vi "Test_ICR.vi"(8 "error in (no error)":errorcluster, 10 "ICR Queue":refnum<queue>, 11 "UI Queue":refnum<queue>) -> (0 "error out":errorcluster)   [LabVIEW 2017]
uses:
  controls/QMH_ICR_Message.ctl
  controls/QMH_ICR_Command.ctl
  controls/QMH_UI_Message.ctl
  controls/QMH_UI_Command.ctl
  controls/HARDWARE_Resources.ctl
  controls/PROCESSING_Inputs.ctl
  controls/QMH_ICR_Cluster.ctl
panel:
  out "Accum Name":string
  in  "PROCESSING  Inputs":T1={"Reference Mass"=300.0939, "Cyclotron Freq"=255.727, "Magnetron Freq"=0.001} caption="DATA Inputs" {"Magnetron Freq" format="%.5g"; "Cyclotron Freq" format="%.5g"; "Reference Mass" format="%.5g"}
  in  "Start":bool
  in  "Stop":bool
  in  "Send Trigger":bool
  out "Total Duration":i32
  out "Number of  Accumulations":i16
  out "Accumulation":i16
  in  "Use Software Trigger":bool=TRUE
  in  "Graph Chooser":T2(radio)=enum."Mass Spectrum"
  out "Remaining Time":string
  out "Spectrum Path":path
  out "Spectrum Prefix":string
  out "Spectrum Name":string
  out "Mass Accumulated":cluster{dbl[], dbl[]}(graph)
  out "Mass Spectrum":cluster{dbl[], dbl[]}(graph)
  out "Frequency Spectrum":cluster{dbl[], dbl[]}(graph)
  out "Signal":cluster{dbl[], dbl[]}(graph)
  in  "HARDWARE Resources":T3={"AO6711 Physical Channels"="Analog/ao0:3", "AO6711 Task Name"="", "AWG5421 Resource Name"="Waveform", "DIGIT 5122 Resource Name"="Digitizer", "HSDIO Resource Name"="Sequencer"}
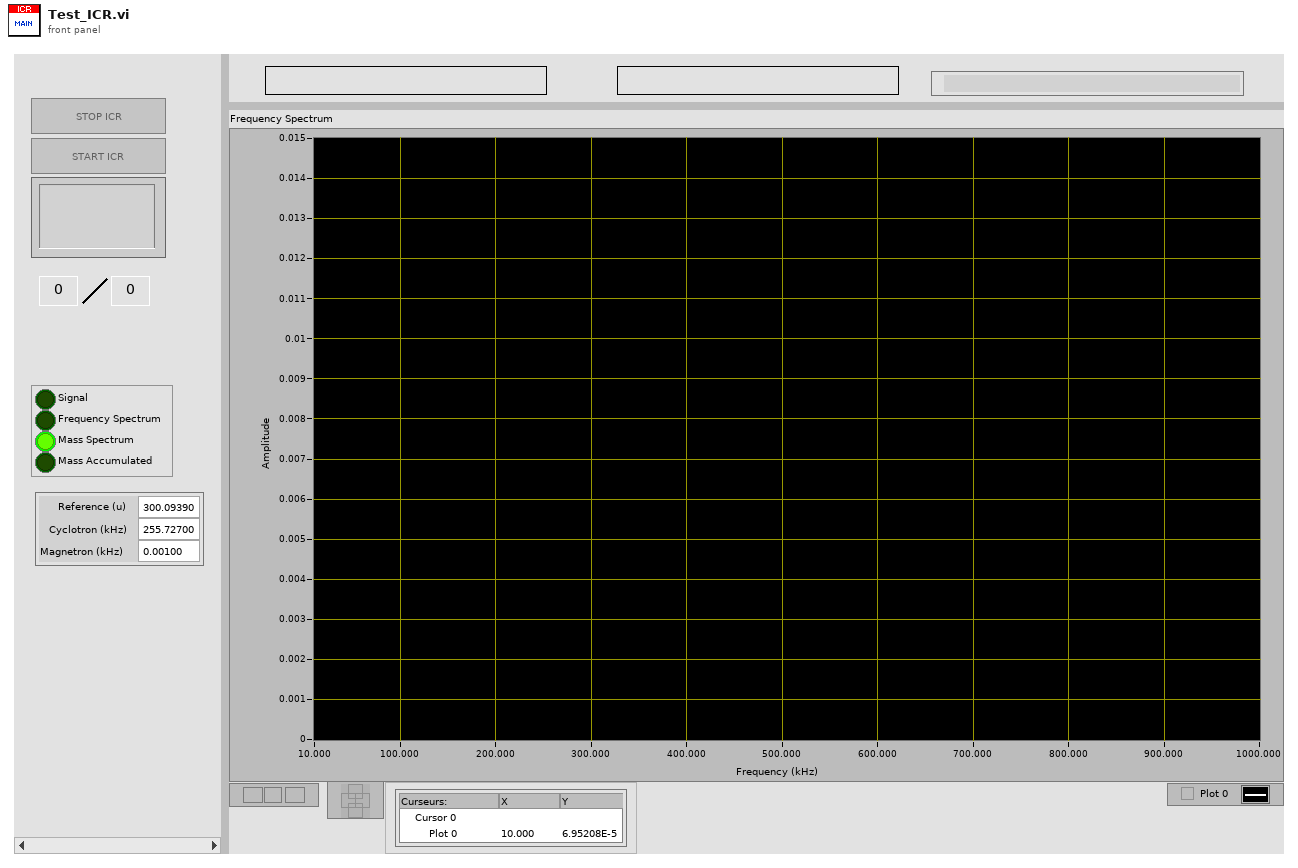
[diagram p1: front panel]
types:
  T1 = typedef "PROCESSING_Inputs.ctl" = cluster{"Reference Mass":dbl, "Cyclotron Freq":dbl, "Magnetron Freq":dbl}
  T2 = enum32{"Signal", "Frequency Spectrum", "Mass Spectrum", "Mass Accumulated"}
  T3 = typedef "HARDWARE_Resources.ctl" = cluster{"AO6711 Physical Channels":tag, "AO6711 Task Name":refnum<k21>, "AWG5421 Resource Name":refnum<k15>, "DIGIT 5122 Resource Name":refnum<k15>, "HSDIO Resource Name":refnum<k15>}
  T4 = typedef "QMH_ICR_Cluster.ctl" = cluster{"Use Software Trigger":refnum<vi>, "Send Trigger":refnum<vi>, "Stop":refnum<vi>, "Start":refnum<vi>, "HARDWARE Resources":refnum<vi>, "Total Duration":refnum<vi>, "Remaining Time":refnum<vi>, "Accumulation":refnum<vi>, "Number of  Accumulations":refnum<vi>, "Graph Chooser":refnum<vi>, "Signal":refnum<vi>, "Frequency Spectrum":refnum<vi>, "Mass Spectrum":refnum<vi>, "Mass Accumulated":refnum<vi>, "Processing":refnum<vi>, "Spectrum Path":refnum<vi>, "Spectrum Prefix":refnum<vi>, "Spectrum Name":refnum<vi>, "Accum Name":refnum<vi>, "Disk Writing Done":refnum<notifier>}
  T5 = typedef "QMH_ICR_Command.ctl" = enum16{"Initialize", "Sequence Setup", "ICR Start", "ICR Stop", "Hardware Setup", "Next Accumulation", "Waiting for Trigger", "Sequence Started", "Sequence Finished", "Writing Data", "Hardware Reset", "Exit"}
  T6 = typedef "QMH_UI_Command.ctl" = enum16{"Initialize", "UI Load", "UI Save", "UI Save As", "UI Change Experiment", "UI Change Voltages", "UI Change Sequence", "UI Change Expert", "Ready to Start", "UI Start", "Waiting for ICR", "UI Exit", "Update Report", "Update ICR Report"}
  T7 = typedef "QMH_ICR_Message.ctl" = cluster{"Command":T5, "Data":variant}
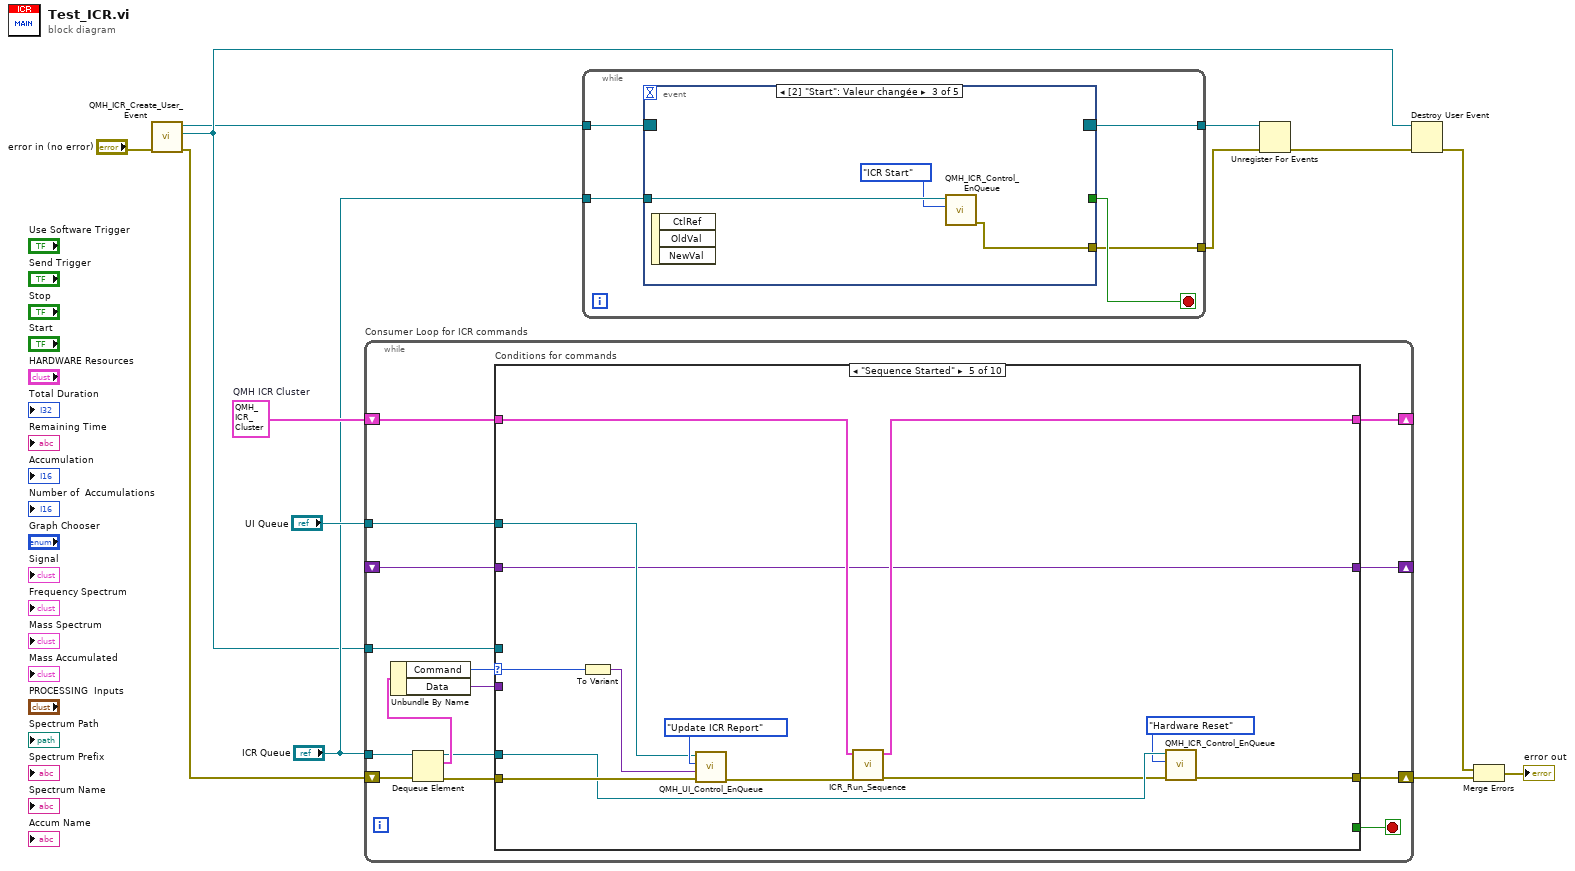
[diagram p0: block diagram]
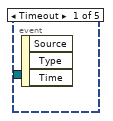
[diagram p2: hidden frame]
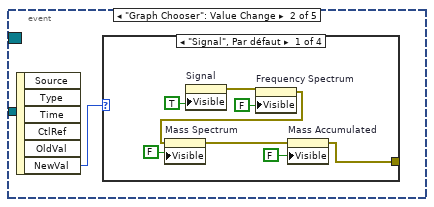
[diagram p3: hidden frame]
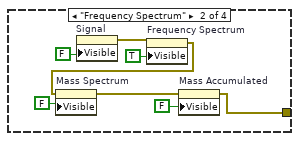
[diagram p4: hidden frame]
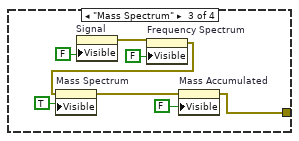
[diagram p5: hidden frame]
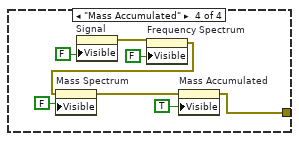
[diagram p6: hidden frame]
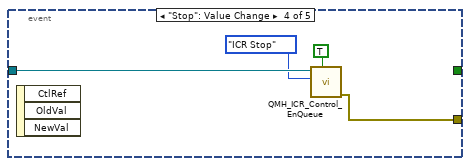
[diagram p7: hidden frame]
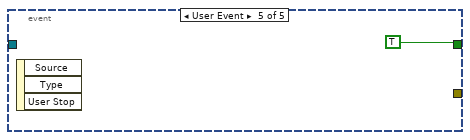
[diagram p8: hidden frame]
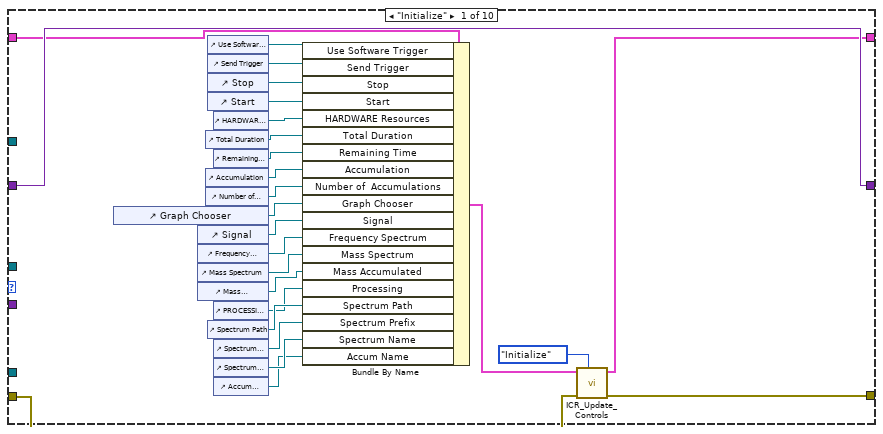
[diagram p9: hidden frame]
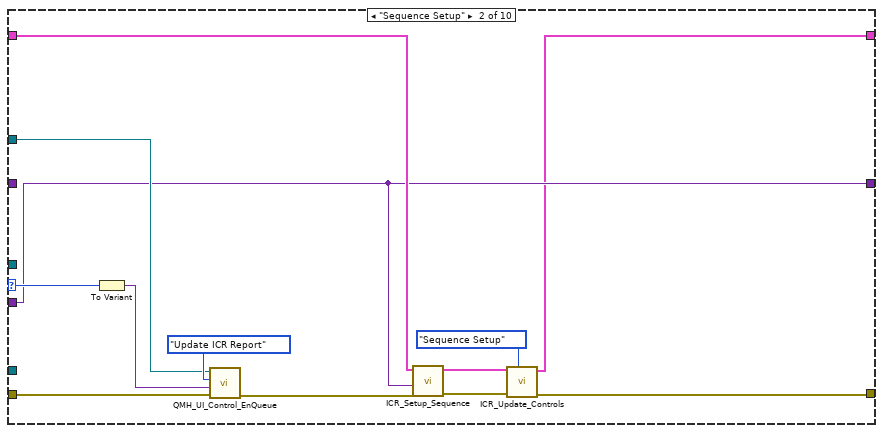
[diagram p10: hidden frame]
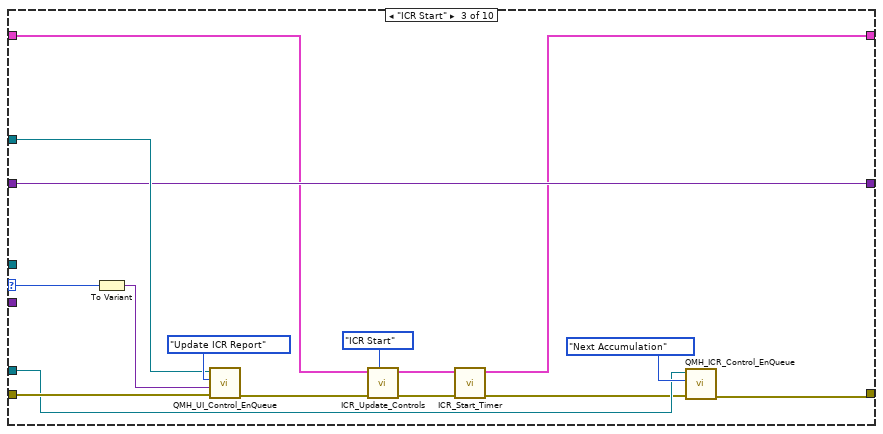
[diagram p11: hidden frame]
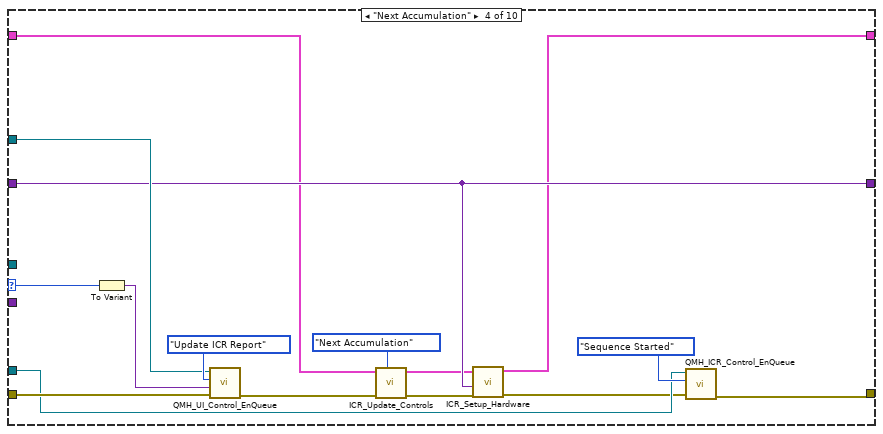
[diagram p12: hidden frame]
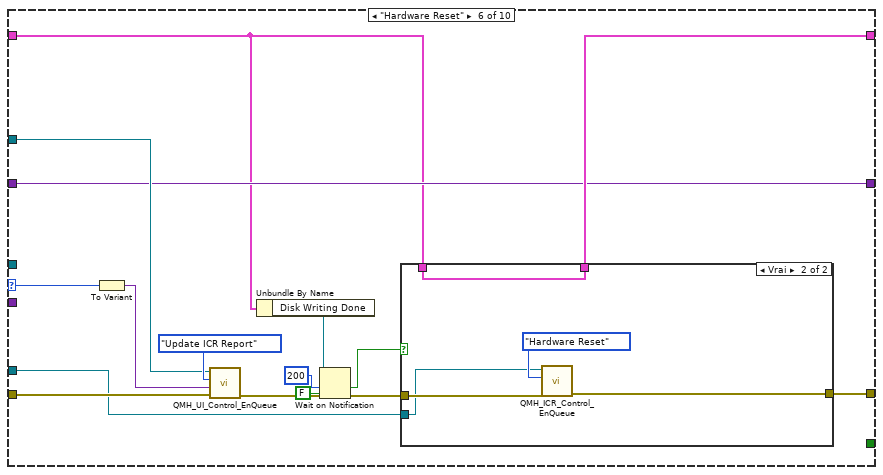
[diagram p13: hidden frame]
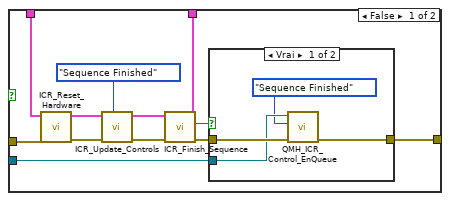
[diagram p14: hidden frame]
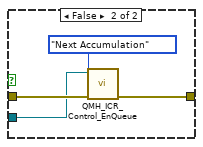
[diagram p15: hidden frame]
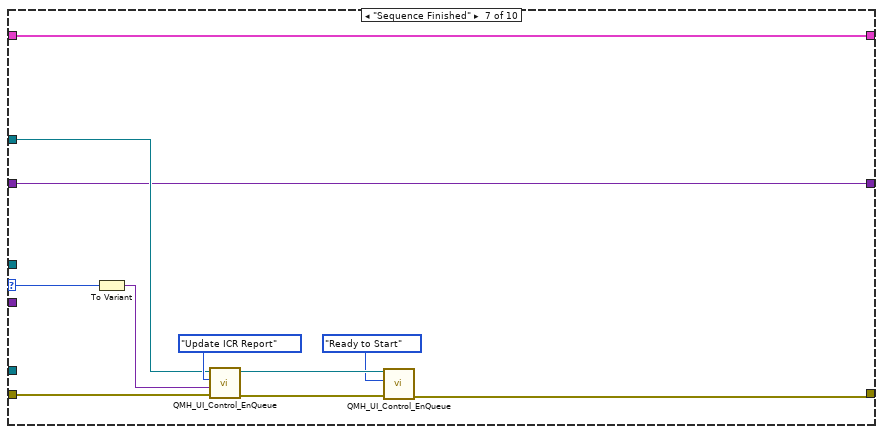
[diagram p16: hidden frame]
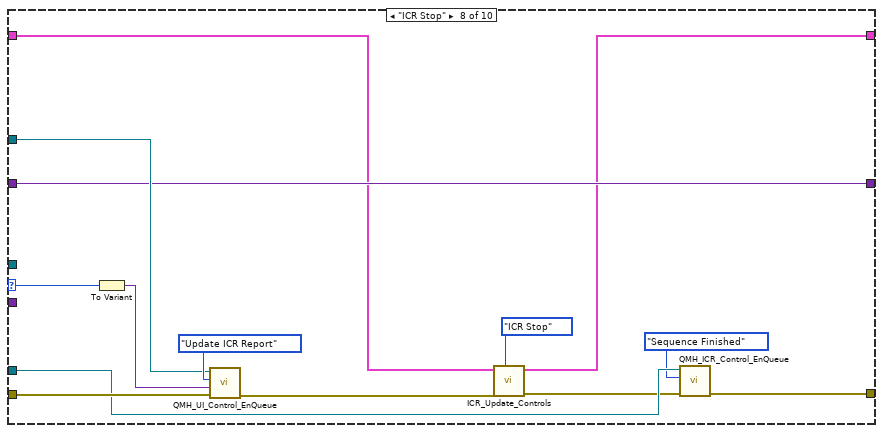
[diagram p17: hidden frame]
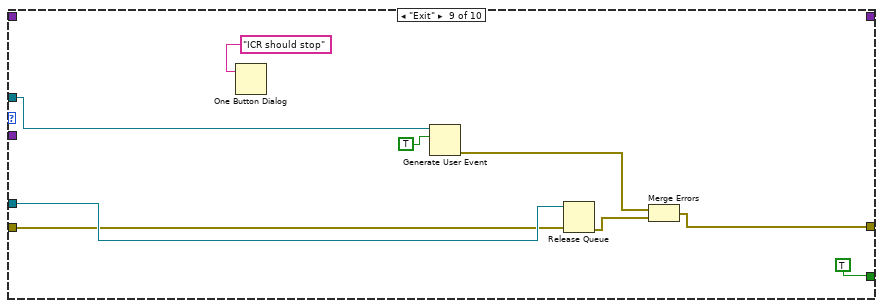
[diagram p18: hidden frame]
diagram:
  w6 = T4 {"Use Software Trigger"=refnum, "Send Trigger"=refnum, "Stop"=refnum, "Start"=refnum, "HARDWARE Resources"=refnum, "Total Duration"=refnum, "Remaining Time"=refnum, "Accumulation"=refnum, "Number of  Accumulations"=refnum, "Graph Chooser"=refnum, "Signal"=refnum, "Frequency Spectrum"=refnum, "Mass Spectrum"=refnum, "Mass Accumulated"=refnum, "Processing"=refnum, "Spectrum Path"=refnum, "Spectrum Prefix"=refnum, "Spectrum Name"=refnum, "Accum Name"=refnum, "Disk Writing Done"=refnum}  # QMH ICR Cluster
  n1 = call "QMH_ICR_Create_User_Event.vi"("error in (no error)"="error in (no error)") -> ("error out"=w11:errorcluster, "User Stop Event"=w2:refnum<user-event>, "Refnum register for events"=w1:refnum<event-registration>)  [unwired: 8 in]
  n2 = while "Consumer Loop for ICR commands" {
    shift-right: [w19] -> w7
    shift-left: w11 -> [w26]
    tunnel: "ICR Queue" -> [w27]
    tunnel: "UI Queue" -> [w21]
    shift-right: [w18] -> _
    shift-left: _ -> [w17]
    tunnel: w2 -> [w16]
    shift-right: [w14] -> _
    shift-left: w6 -> [w15]
    stop <- w20 stop-if-true
    n3 = Dequeue Element(queue=w27, error in (no error)=w26) -> (queue out=w25:refnum<queue>, element=w28:T7, error out=w22:errorcluster)  [unwired: 2 out]
    n4 = Unbundle By Name(w28) -> ("Command"=w24:T5, "Data"=w23:variant)
    n5 = case "Conditions for commands" shown="\"Sequence Started\"" w24 {
      selector: w24 -> [_ w64 w80 w96 w109 w125 w161 w175 _ _]
      tunnel: w25 -> [_ _ w76 w92 w106 w122 _ w172 w187 _]
      tunnel: w23 -> [_ w60 _ _ _ _ _ _ _ _]
      tunnel: w22 -> [w49 w63 w79 w95 w108 w124 w160 w174 w179 _]
      tunnel: w21 -> [_ w65 w81 w97 w110 w126 w162 w176 _ _]
      tunnel: [_ _ _ _ _ _ _ _ TRUE _] -> w20
      tunnel: [w47 w55 w77 w93 w107 w123 w155 w173 w180 _] -> w19
      tunnel: [w54 w60 w75 w91 w101 w120 w159 w171 _ _] -> w18
      tunnel: w17 -> [w54 _ w75 w91 w101 w120 w159 w171 _ _]
      tunnel: w16 -> [_ _ _ _ _ _ _ _ w184 _]
      tunnel: w15 -> [w46 w61 w71 w88 w104 w119 w154 w169 _ _]
      tunnel: [w48 w57 w69 w86 w102 w121 w154 w167 _ _] -> w14
      frame "Initialize" {
        n6 = control-ref of="Graph Chooser"() -> (w50:refnum<vi>)
        n7 = control-ref of="Signal"() -> (w29:refnum<vi>)
        n8 = control-ref of="Frequency Spectrum"() -> (w51:refnum<vi>)
        n9 = control-ref of="Mass Spectrum"() -> (w52:refnum<vi>)
        n10 = control-ref of="Mass Accumulated"() -> (w40:refnum<vi>)
        n11 = control-ref of="Total Duration"() -> (w34:refnum<vi>)
        n12 = control-ref of="Accumulation"() -> (w31:refnum<vi>)
        n13 = control-ref of="Number of  Accumulations"() -> (w30:refnum<vi>)
        n14 = control-ref of="Use Software Trigger"() -> (w53:refnum<vi>)
        n15 = control-ref of="Send Trigger"() -> (w38:refnum<vi>)
        n16 = control-ref of="Stop"() -> (w37:refnum<vi>)
        n17 = control-ref of="Start"() -> (w36:refnum<vi>)
        n18 = control-ref of="Spectrum Path"() -> (w43:refnum<vi>)
        n19 = control-ref of="HARDWARE Resources"() -> (w35:refnum<vi>)
        n20 = control-ref of="Remaining Time"() -> (w33:refnum<vi>)
        n21 = control-ref of="PROCESSING  Inputs"() -> (w39:refnum<vi>)
        n22 = control-ref of="Spectrum Prefix"() -> (w42:refnum<vi>)
        n23 = control-ref of="Spectrum Name"() -> (w41:refnum<vi>)
        n24 = control-ref of="Accum Name"() -> (w32:refnum<vi>)
        n25 = Bundle By Name(cluster=w46, "Use Software Trigger"=w53, "Send Trigger"=w38, "Stop"=w37, "Start"=w36, "HARDWARE Resources"=w35, "Total Duration"=w34, "Remaining Time"=w33, "Accumulation"=w31, "Number of  Accumulations"=w30, "Graph Chooser"=w50, "Signal"=w29, "Frequency Spectrum"=w51, "Mass Spectrum"=w52, "Mass Accumulated"=w40, "Processing"=w39, "Spectrum Path"=w43, "Spectrum Prefix"=w42, "Spectrum Name"=w41, "Accum Name"=w32) -> (w45:T4)
        n26 = call "ICR_Update_Controls.vi"("Command"=QMH_ICR_Command."Initialize", "error in (no error)"=w49, "QMH ICR Cluster"=w45) -> ("error out"=w47:errorcluster, "QMH ICR Cluster"=w48:T4)  [unwired: 7 in]
      }
      frame "Sequence Setup" {
        n27 = To Variant(anything=w64) -> (Variant=w66:variant)
        n28 = call "QMH_UI_Control_EnQueue.vi"("error in (no error)"=w63, "Variant"=w66, "Command"=QMH_UI_Command."Update ICR Report", "UI Queue"=w65) -> ("error out"=w62:errorcluster)  [unwired: 6 in, 1 out]
        n29 = call "ICR_Setup_Sequence.vi"("error in (no error)"=w62, "QMH UI Cluster"=w60, "QMH ICR Cluster"=w61) -> ("error out"=w59:errorcluster, "QMH ICR Cluster"=w58:T4)  [unwired: 7 in]
        n30 = call "ICR_Update_Controls.vi"("Command"=QMH_ICR_Command."Sequence Setup", "error in (no error)"=w59, "QMH ICR Cluster"=w58) -> ("error out"=w55:errorcluster, "QMH ICR Cluster"=w57:T4)  [unwired: 7 in]
      }
      frame "ICR Start" {
        n31 = To Variant(anything=w80) -> (Variant=w82:variant)
        n32 = call "QMH_UI_Control_EnQueue.vi"("error in (no error)"=w79, "Variant"=w82, "Command"=QMH_UI_Command."Update ICR Report", "UI Queue"=w81) -> ("error out"=w74:errorcluster)  [unwired: 6 in, 1 out]
        n33 = call "ICR_Update_Controls.vi"("Command"=QMH_ICR_Command."ICR Start", "error in (no error)"=w74, "QMH ICR Cluster"=w71) -> ("error out"=w73:errorcluster, "QMH ICR Cluster"=w70:T4)  [unwired: 7 in]
        n34 = call "ICR_Start_Timer.vi"("error in (no error)"=w73, "QMH ICR Cluster"=w70) -> ("error out"=w68:errorcluster, "QMH ICR Cluster"=w69:T4)  [unwired: 8 in]
        n35 = call "QMH_ICR_Control_EnQueue.vi"("error in (no error)"=w68, "Command"=QMH_ICR_Command."Next Accumulation", "ICR Queue"=w76) -> ("error out"=w77:errorcluster)  [unwired: 7 in, 1 out]
      }
      frame "Next Accumulation" {
        n36 = To Variant(anything=w96) -> (Variant=w98:variant)
        n37 = call "QMH_UI_Control_EnQueue.vi"("error in (no error)"=w95, "Variant"=w98, "Command"=QMH_UI_Command."Update ICR Report", "UI Queue"=w97) -> ("error out"=w90:errorcluster)  [unwired: 6 in, 1 out]
        n38 = call "ICR_Update_Controls.vi"("Command"=QMH_ICR_Command."Next Accumulation", "error in (no error)"=w90, "QMH ICR Cluster"=w88) -> ("error out"=w89:errorcluster, "QMH ICR Cluster"=w87:T4)  [unwired: 7 in]
        n39 = call "ICR_Setup_Hardware.vi"("error in (no error)"=w89, "QMH UI Cluster"=w91, "QMH ICR Cluster"=w87) -> ("error out"=w85:errorcluster, "QMH ICR Cluster"=w86:T4)  [unwired: 7 in]
        n40 = call "QMH_ICR_Control_EnQueue.vi"("error in (no error)"=w85, "Command"=QMH_ICR_Command."Sequence Started", "ICR Queue"=w92) -> ("error out"=w93:errorcluster)  [unwired: 7 in, 1 out]
      }
      frame "Sequence Started" {
        n41 = To Variant(anything=w109) -> (Variant=w111:variant)
        n42 = call "QMH_UI_Control_EnQueue.vi"("error in (no error)"=w108, "Variant"=w111, "Command"=QMH_UI_Command."Update ICR Report", "UI Queue"=w110) -> ("error out"=w105:errorcluster)  [unwired: 6 in, 1 out]
        n43 = call "ICR_Run_Sequence.vi"("error in (no error)"=w105, "QMH ICR Cluster"=w104) -> ("error out"=w103:errorcluster, "QMH ICR Cluster"=w102:T4)  [unwired: 8 in]
        n44 = call "QMH_ICR_Control_EnQueue.vi"("error in (no error)"=w103, "Command"=QMH_ICR_Command."Hardware Reset", "ICR Queue"=w106) -> ("error out"=w107:errorcluster)  [unwired: 7 in, 1 out]
      }
      frame "Hardware Reset" {
        n45 = To Variant(anything=w125) -> (Variant=w127:variant)
        n46 = call "QMH_UI_Control_EnQueue.vi"("error in (no error)"=w124, "Variant"=w127, "Command"=QMH_UI_Command."Update ICR Report", "UI Queue"=w126) -> ("error out"=w116:errorcluster)  [unwired: 6 in, 1 out]
        n47 = Unbundle By Name(w119) -> ("Disk Writing Done"=w118:refnum<notifier>)
        n48 = Wait on Notification(notifier=w118, ignore previous (F)=FALSE ("ignorer les précédents (F)"), timeout in ms (-1)=200 ("timeout en ms (-1)"), error in (no error)=w116) -> (timed out?=w114:bool, error out=w115:errorcluster)  [unwired: 2 out]
        n49 = case shown="Vrai" w114 {
          tunnel: [w140 w150] -> w123
          tunnel: w122 -> [w139 w151]
          tunnel: [w137 w149] -> w121
          tunnel: w119 -> [w130 w149]
          tunnel: w115 -> [w129 w152]
          frame False {
            n50 = call "ICR_Reset_Hardware.vi"("error in (no error)"=w129, "QMH ICR Cluster"=w130) -> ("error out"=w133:errorcluster, "QMH ICR Cluster"=w135:T4)  [unwired: 8 in]
            n51 = call "ICR_Update_Controls.vi"("Command"=QMH_ICR_Command."Sequence Finished", "error in (no error)"=w133, "QMH ICR Cluster"=w135) -> ("error out"=w132:errorcluster, "QMH ICR Cluster"=w134:T4)  [unwired: 7 in]
            n52 = call "ICR_Finish_Sequence.vi"("error in (no error)"=w132, "QMH ICR Cluster"=w134) -> ("error out"=w138:errorcluster, "Is Finished ?"=w136:bool, "QMH ICR Cluster"=w137:T4)  [unwired: 7 in]
            n53 = case shown="Vrai" w136 {
              tunnel: w138 -> [w144 w148]
              tunnel: [w143 w147] -> w140
              tunnel: w139 -> [w142 w146]
              frame True {
                n54 = call "QMH_ICR_Control_EnQueue.vi"("error in (no error)"=w144, "Command"=QMH_ICR_Command."Sequence Finished", "ICR Queue"=w142) -> ("error out"=w143:errorcluster)  [unwired: 7 in, 1 out]
              }
              frame False {
                n55 = call "QMH_ICR_Control_EnQueue.vi"("error in (no error)"=w148, "Command"=QMH_ICR_Command."Next Accumulation", "ICR Queue"=w146) -> ("error out"=w147:errorcluster)  [unwired: 7 in, 1 out]
              }
            }
          }
          frame True {
            n56 = call "QMH_ICR_Control_EnQueue.vi"("error in (no error)"=w152, "Command"=QMH_ICR_Command."Hardware Reset", "ICR Queue"=w151) -> ("error out"=w150:errorcluster)  [unwired: 7 in, 1 out]
          }
        }
      }
      frame "Sequence Finished" {
        n57 = To Variant(anything=w161) -> (Variant=w163:variant)
        n58 = call "QMH_UI_Control_EnQueue.vi"("error in (no error)"=w160, "Variant"=w163, "Command"=QMH_UI_Command."Update ICR Report", "UI Queue"=w162) -> ("error out"=w158:errorcluster, "UI Queue"=w157:refnum<queue>)  [unwired: 6 in]
        n59 = call "QMH_UI_Control_EnQueue.vi"("error in (no error)"=w158, "Command"=QMH_UI_Command."Ready to Start", "UI Queue"=w157) -> ("error out"=w155:errorcluster)  [unwired: 7 in, 1 out]
      }
      frame "ICR Stop" {
        n60 = To Variant(anything=w175) -> (Variant=w177:variant)
        n61 = call "QMH_UI_Control_EnQueue.vi"("error in (no error)"=w174, "Variant"=w177, "Command"=QMH_UI_Command."Update ICR Report", "UI Queue"=w176) -> ("error out"=w168:errorcluster)  [unwired: 6 in, 1 out]
        n62 = call "ICR_Update_Controls.vi"("Command"=QMH_ICR_Command."ICR Stop", "error in (no error)"=w168, "QMH ICR Cluster"=w169) -> ("error out"=w165:errorcluster, "QMH ICR Cluster"=w167:T4)  [unwired: 7 in]
        n63 = call "QMH_ICR_Control_EnQueue.vi"("error in (no error)"=w165, "Command"=QMH_ICR_Command."Sequence Finished", "ICR Queue"=w172) -> ("error out"=w173:errorcluster)  [unwired: 7 in, 1 out]
      }
      frame "Exit" {
        n64 = One Button Dialog(message="ICR should stop") -> ()  [unwired: 1 in, 1 out]
        n65 = Generate User Event(user event=w184, event data cluster=TRUE ("données d'événement")) -> (error out=w182:errorcluster)  [unwired: 2 in, 1 out]
        n66 = Release Queue(queue=w187, error in (no error)=w179) -> (error out=w181:errorcluster)  [unwired: 1 in, 2 out]
        n67 = Merge Errors(w182, w181) -> (w180:errorcluster)
      }
      frame Default {
      }
    }
  }
  n68 = while {
    tunnel: [w191] -> w10
    tunnel: [w190] -> w9
    tunnel: "ICR Queue" -> [w189]
    tunnel: w1 -> [w188]
    stop <- w192 stop-if-true
    n69 = event shown="[2] \"Start\": Valeur changée" {
      selector: w188 -> [_ _ _ _ _]
      dyn-events: [_ _ _ _ _] -> w191
      timeout: _ -> [_ _ _ _ _]
      tunnel: [_ _ _ _ TRUE] -> w192
      tunnel: [_ _ w228 w232 _] -> w190
      tunnel: w189 -> [_ _ w227 w231 _]
      event Timeout {
        n70 = event-data() -> ()  [unwired: 1 in, 3 out]
      }
      event "Graph Chooser": Value Change {
        n71 = event-data() -> ("NewVal"=w193:T2)  [unwired: 1 in, 5 out]
        n72 = case shown="\"Signal\", Par défaut" w193 {
          tunnel: [w194 w205 w213 w218] -> _
          frame "Signal", Default {
            n73 = property on="Signal" class="GraphXY (strict)"("Visible"=TRUE) -> (error out=w197:errorcluster)  [unwired: 2 in, 1 out]
            n74 = property on="Frequency Spectrum" class="GraphXY (strict)"(error in=w197, "Visible"=FALSE) -> (error out=w196:errorcluster)  [unwired: 1 in, 1 out]
            n75 = property on="Mass Spectrum" class="GraphXY (strict)"(error in=w196, "Visible"=FALSE) -> (error out=w195:errorcluster)  [unwired: 1 in, 1 out]
            n76 = property on="Mass Accumulated" class="GraphXY (strict)"(error in=w195, "Visible"=FALSE) -> (error out=w194:errorcluster)  [unwired: 1 in, 1 out]
          }
          frame "Frequency Spectrum" {
            n77 = property on="Signal" class="GraphXY (strict)"("Visible"=FALSE) -> (error out=w202:errorcluster)  [unwired: 2 in, 1 out]
            n78 = property on="Frequency Spectrum" class="GraphXY (strict)"(error in=w202, "Visible"=TRUE) -> (error out=w203:errorcluster)  [unwired: 1 in, 1 out]
            n79 = property on="Mass Spectrum" class="GraphXY (strict)"(error in=w203, "Visible"=FALSE) -> (error out=w204:errorcluster)  [unwired: 1 in, 1 out]
            n80 = property on="Mass Accumulated" class="GraphXY (strict)"(error in=w204, "Visible"=FALSE) -> (error out=w205:errorcluster)  [unwired: 1 in, 1 out]
          }
          frame "Mass Spectrum" {
            n81 = property on="Signal" class="GraphXY (strict)"("Visible"=FALSE) -> (error out=w210:errorcluster)  [unwired: 2 in, 1 out]
            n82 = property on="Frequency Spectrum" class="GraphXY (strict)"(error in=w210, "Visible"=FALSE) -> (error out=w211:errorcluster)  [unwired: 1 in, 1 out]
            n83 = property on="Mass Spectrum" class="GraphXY (strict)"(error in=w211, "Visible"=TRUE) -> (error out=w212:errorcluster)  [unwired: 1 in, 1 out]
            n84 = property on="Mass Accumulated" class="GraphXY (strict)"(error in=w212, "Visible"=FALSE) -> (error out=w213:errorcluster)  [unwired: 1 in, 1 out]
          }
          frame "Mass Accumulated" {
            n85 = property on="Signal" class="GraphXY (strict)"("Visible"=FALSE) -> (error out=w221:errorcluster)  [unwired: 2 in, 1 out]
            n86 = property on="Frequency Spectrum" class="GraphXY (strict)"(error in=w221, "Visible"=FALSE) -> (error out=w220:errorcluster)  [unwired: 1 in, 1 out]
            n87 = property on="Mass Spectrum" class="GraphXY (strict)"(error in=w220, "Visible"=FALSE) -> (error out=w219:errorcluster)  [unwired: 1 in, 1 out]
            n88 = property on="Mass Accumulated" class="GraphXY (strict)"(error in=w219, "Visible"=TRUE) -> (error out=w218:errorcluster)  [unwired: 1 in, 1 out]
          }
        }
      }
      event "Start": Value Change {
        n89 = event-data() -> ()  [unwired: 1 in, 3 out]
        n90 = call "QMH_ICR_Control_EnQueue.vi"("Command"=QMH_ICR_Command."ICR Start", "ICR Queue"=w227) -> ("error out"=w228:errorcluster)  [unwired: 8 in, 1 out]
      }
      event "Stop": Value Change {
        n91 = event-data() -> ()  [unwired: 1 in, 3 out]
        n92 = call "QMH_ICR_Control_EnQueue.vi"("Last ?"=TRUE, "Command"=QMH_ICR_Command."ICR Stop", "ICR Queue"=w231) -> ("error out"=w232:errorcluster)  [unwired: 7 in, 1 out]
      }
      event User Event {
        n93 = event-data() -> ()  [unwired: 1 in, 3 out]
      }
    }
  }
  n94 = Unregister For Events(event registration refnum=w10, error in=w9) -> (error out=w4:errorcluster)
  n95 = Destroy User Event(user event=w2, error in=w4) -> (error out=w3:errorcluster)
  n96 = Merge Errors(w3, w7) -> (→"error out":errorcluster)
